vi "Get Owning Path Default Value.vi"(0 "Vector Abstract Path Group in":refnum<class "Vector Abstract Path Group.lvclass">, 11 "error in (no error)":errorcluster) -> (4 "Vector Abstract Path Group out":refnum<class "Vector Abstract Path Group.lvclass">, 6 "Path":refnum<class "Path.lvclass">, 15 "error out":errorcluster)   [LabVIEW 2023, in "RFFixtureCharact.Public.lvlib" / "Vector Abstract Path Group.lvclass"]
uses:
  Vector Abstract Path Group.lvclass
  Vector Abstract Path Group.lvclass/Vector Abstract Path Group.ctl
  Common/Base Classes/Path/Path.lvclass
  Vector Abstract Path/Vector Abstract Path.lvclass
  C:/rfcal/AuxTools/STSRFFixtureCharactUtility/Source/Code Modules/Common/Base Classes/Path/Path.lvclass
  C:/rfcal/AuxTools/STSRFFixtureCharactUtility/Source/Code Modules/Fixture/Public/Base Classes/Vector/Vector Abstract Path/Vector Abstract Path.lvclass
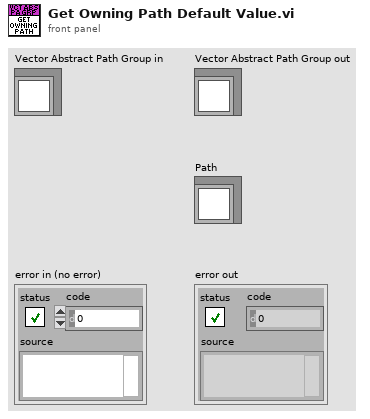
[diagram p1: front panel]
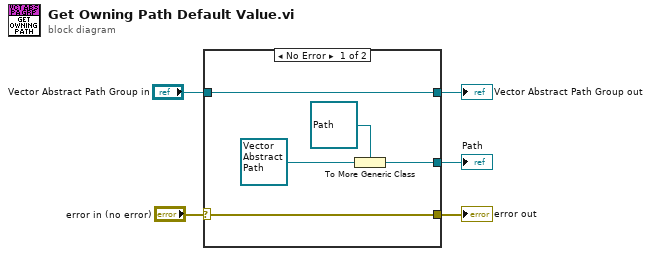
[diagram p0: block diagram]
diagram:
  n1 = case shown="No Error" "error in (no error)" {
    selector: "error in (no error)" -> [w9 w12]
    tunnel: [w9 w12] -> w1
    tunnel: [w10 w11] -> w4
    tunnel: "Vector Abstract Path Group in" -> [w10 w11]
    tunnel: [w7 _] -> w3
    frame No Error {
      n2 = To More Generic Class(target class=refnum<class "Path.lvclass"> refnum ("Path"), reference=refnum<class "Vector Abstract Path.lvclass"> refnum ("RFFixtureCharact.Public.lvlib:Vector Abstract Path.lvclass")) -> (generic class reference=w7:refnum<class "Path.lvclass">)
    }
    frame Error {
    }
  }
  "error out" <- w1
  "Vector Abstract Path Group out" <- w4
  "Path" <- w3
